vi "Read Data.vi"(8 "error in (no error)":errorcluster, 11 "Device in":refnum<class "Cryo-Con-22C.lvclass">) -> (0 "error out":errorcluster, 2 "Data":waveform(dbl)[](array[waveform]), 3 "Device out":refnum<class "Cryo-Con-22C.lvclass">)   [LabVIEW 2015, in "Cryo-Con-22C.lvclass"]
uses:
  Cryo-Con-22C.lvclass
  Cryo-Con Front Panel Data.ctl
  Cryo-con Heater Ranges.ctl
  Cry-Con Loop Type.ctl
  OO Devices/Device/Read Control Panel Loaded.vi
  Instrument/Read VISA Resource.vi
  OO Devices/Device/Read Controls Snapshot.vi
  Instrument/Write VISA Resource.vi
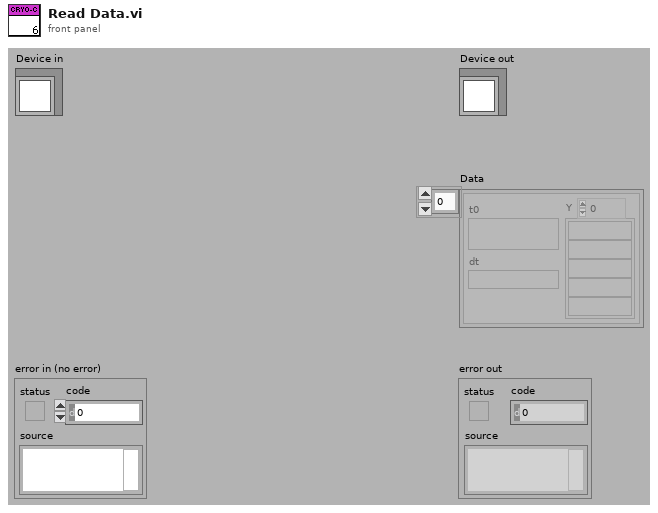
[diagram p1: front panel]
types:
  T1 = typedef "Cryo-Con Front Panel Data.ctl" = cluster{"Channels to measure":string[], "Record heater":bool, "Set point":dbl, "Heater Range":T2, "Control":bool, "Loop type":T3, "Ramp rate,\n K/min":dbl, "Control Channel":string, "P":dbl, "I":dbl, "D":dbl, "Manual %":u16}
  T2 = typedef "Cryo-con Heater Ranges.ctl" = enum16{"25W", "2.5W", "0.25W"}
  T3 = typedef "Cry-Con Loop Type.ctl" = enum16{"Off", "PID", "Manual", "PID Table", "PID Ramp", "PID Table Ramp"}
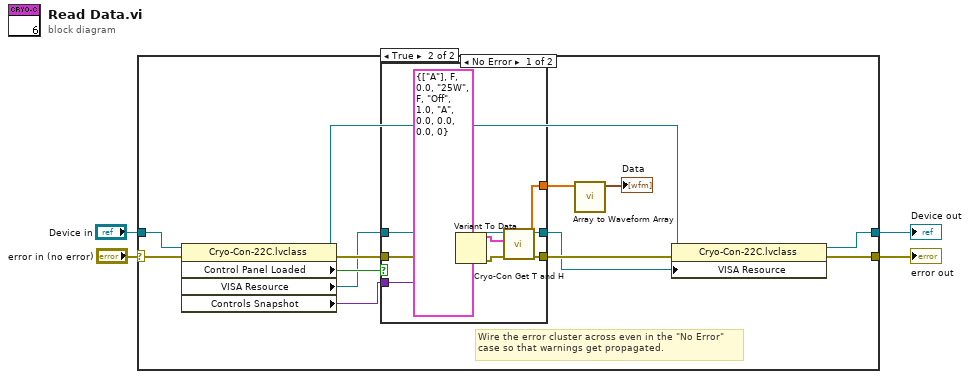
[diagram p0: block diagram]
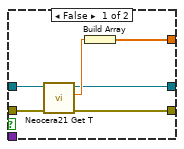
[diagram p2: hidden frame]
diagram:
  n1 = case shown="No Error" "error in (no error)" {
    selector: "error in (no error)" -> [w9 w34]
    tunnel: [w15 w34] -> w3
    tunnel: [w17 w33] -> w1
    tunnel: "Device in" -> [w8 w33]
    frame No Error {
      # "Wire the error cluster across even in the \"No Error\"\ncase so that warnings get propagated."
      n2 = property class="Cryo-Con-22C.lvclass"(reference=w8, error in=w9) -> (reference out=w5:refnum<class "Cryo-Con-22C.lvclass">, error out=w12:errorcluster, "Control Panel Loaded"=w11:bool, "VISA Resource"=w10:refnum<visa-resource-name>, "Controls Snapshot"=w6:variant)
      n3 = case shown="True" w11 {
        tunnel: [w18 w32] -> w7
        tunnel: [w23 w31] -> w16
        tunnel: w10 -> [w21 w30]
        tunnel: [w19 w29] -> w13
        tunnel: w12 -> [w22 w24]
        tunnel: w6 -> [_ w25]
        frame False {
          n4 = call "Neocera21 Get T.vi"("error in (no error)"=w22, "VISA Resource Name"=w21) -> ("error out"=w23:errorcluster, "Temperature"=w20:dbl, "VISA Resource Name Out"=w18:refnum<visa-resource-name>)  [unwired: 6 in, 1 out]
          n5 = Build Array(w20) -> (w19:dbl[])
        }
        frame True {
          n6 = Variant To Data(error in=w24, type=T1 {"Channels to measure"=["A"], "Record heater"=FALSE, "Set point"=0.0, "Heater Range"=enum."25W", "Control"=FALSE, "Loop type"=enum."Off", "Ramp rate,\n K/min"=1.0, "Control Channel"="A", "P"=0.0, "I"=0.0, "D"=0.0, "Manual %"=0} ("Private data"), Variant=w25) -> (data=w27:T1, error out=w26:errorcluster)
          n7 = call "Cryo-Con Get T and H.vi"("error in (no error)"=w26, "Private data"=w27, "VISA Resource Name"=w30) -> ("error out"=w31:errorcluster, "Data out"=w29:dbl[], "VISA Resource Name Out"=w32:refnum<visa-resource-name>)  [unwired: 4 in, 2 out]
        }
      }
      n8 = call "Array to Waveform Array.vi"("Array"=w13) -> ("Waveform"=→"Data":waveform(dbl)[])  [unwired: 10 in]
      n9 = property class="Cryo-Con-22C.lvclass"(reference=w5, error in=w16, "VISA Resource"=w7) -> (reference out=w17:refnum<class "Cryo-Con-22C.lvclass">, error out=w15:errorcluster)
    }
    frame Error {
    }
  }
  "error out" <- w3
  "Device out" <- w1
